vi "Create Oneof Class Converter.vi"(7 "Oneof Container Name":string, 8 "error in (no error)":errorcluster, 9 "Is in Oneof":bool, 10 "LVClassLibrary in":refnum<vi>, 11 "Library":refnum<vi>) -> (0 "error out":errorcluster, 2 "LVClassLibrary out":refnum<vi>, 3 "Library out":refnum<vi>)   [LabVIEW 2019, in "gRPC Template Creation Utility.lvlib"]
uses:
  gRPC Template Creation Utility.lvlib
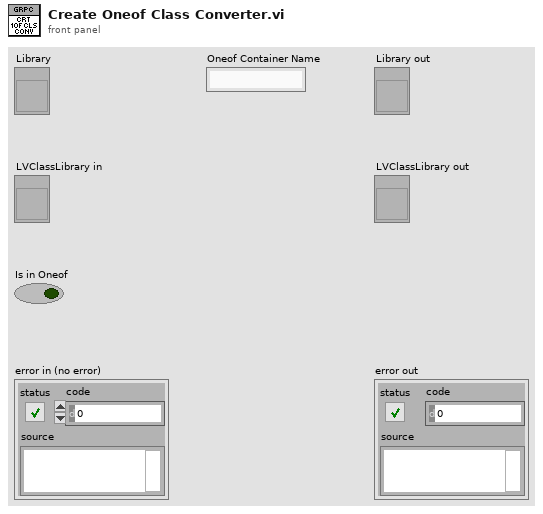
[diagram p1: front panel]
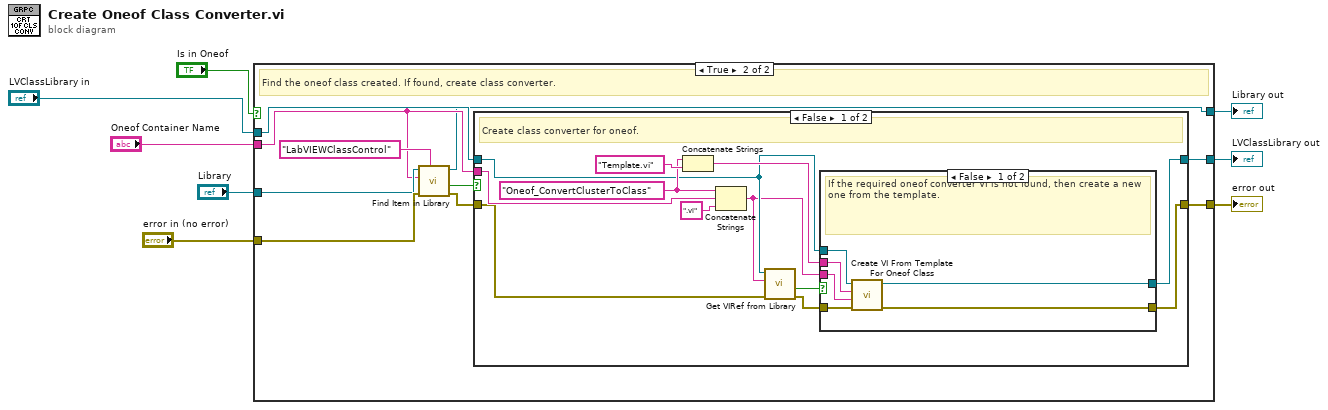
[diagram p0: block diagram]
diagram:
  n1 = case shown="True" "Is in Oneof" {
    tunnel: "Oneof Container Name" -> [_ w14]
    tunnel: "error in (no error)" -> [w11 w21]
    tunnel: "Library" -> [w10 w20]
    tunnel: "LVClassLibrary in" -> [w9 w19]
    tunnel: [w11 w15] -> w7
    tunnel: [w10 w13] -> w2
    tunnel: [w9 w12] -> w1
    frame False {
    }
    frame True {
      # "Find the oneof class created. If found, create class converter."
      n2 = call "Find Item in Library.vi"("Item Type"="LabVIEWClassControl", "error in (no error)"=w21, "Item Name"=w14, "Library item in"=w20) -> ("error out"=w17:errorcluster, "Found?"=w16:bool, "Library item out"=w13:refnum<vi>)  [unwired: 4 in, 1 out]
      n3 = case shown="False" w16 {
        tunnel: w19 -> [w27 w42]
        tunnel: w17 -> [w25 w43]
        tunnel: [w28 w43] -> w15
        tunnel: w14 -> [w32 _]
        tunnel: [w22 w42] -> w12
        frame False {
          w29 = "Oneof_ConvertClusterToClass" ("Name")
          # "Create class converter for oneof."
          n4 = Concatenate Strings(w29, "Template.vi" ("string")) -> (w30:string)
          n5 = Concatenate Strings(w29, w32, ".vi" ("string")) -> (w26:string)
          n6 = call "Get VIRef from Library.vi"("error in (no error)"=w25, "Item Name"=w26, "Library"=w27) -> ("error out"=w24:errorcluster, "Found ?"=w23:bool)  [unwired: 5 in, 2 out]
          n7 = case shown="False" w23 {
            tunnel: w30 -> [w39 _]
            tunnel: [w38 w41] -> w28
            tunnel: w27 -> [w37 w40]
            tunnel: w26 -> [w36 _]
            tunnel: w24 -> [w35 w41]
            tunnel: [w34 w40] -> w22
            frame False {
              # "If the required oneof converter VI is not found, then create a new one from the template."
              n8 = call "Create VI From Template For Oneof Class.vi"("error in (no error)"=w35, "VI name"=w36, "template name"=w39, "LVClassLibrary in"=w37) -> ("error out"=w38:errorcluster, "LVClassLibrary out"=w34:refnum<vi>)  [unwired: 5 in, 1 out]
            }
            frame True {
              # "If the oneof converter already exists, then do nothing."
            }
          }
        }
        frame True {
        }
      }
    }
  }
  "error out" <- w7
  "Library out" <- w2
  "LVClassLibrary out" <- w1
